vi "Check For License.vi"(8 "error in (no error)":errorcluster, 11 "VI Reference":refnum<vi>) -> (0 "Error Out":errorcluster, 2 "License Type":T1=enum."Professional", 3 "Valid License?":bool)   [LabVIEW 2022 SP3]
uses:
  <userlib>/_MGI/Error Reporter/MGI Error Reporter Base/MGI Error Reporter Base.lvclass
  Controls/License Types.ctl
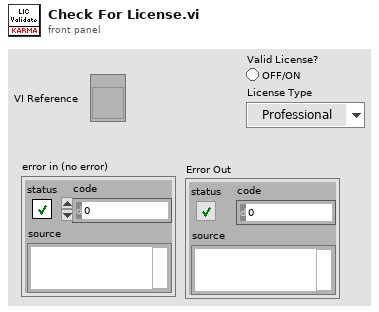
[diagram p1: front panel]
types:
  T1 = typedef "License Types.ctl" = enum16{"Evaluation", "Professional"}
  T2 = typedef "Paths.ctl" = cluster{"Configuration":path, "Event Logs":path, "Error Logs":path, "Configuration.ini":path}
  T3 = typedef "License File Data.ctl" = cluster{"Computer ID":string, "License Requested Date":string, "License Generated Date":string, "License Type":T1, "Evaluation Period":string, "License Generated Time":timestamp, "Sensor Serial Number":string}
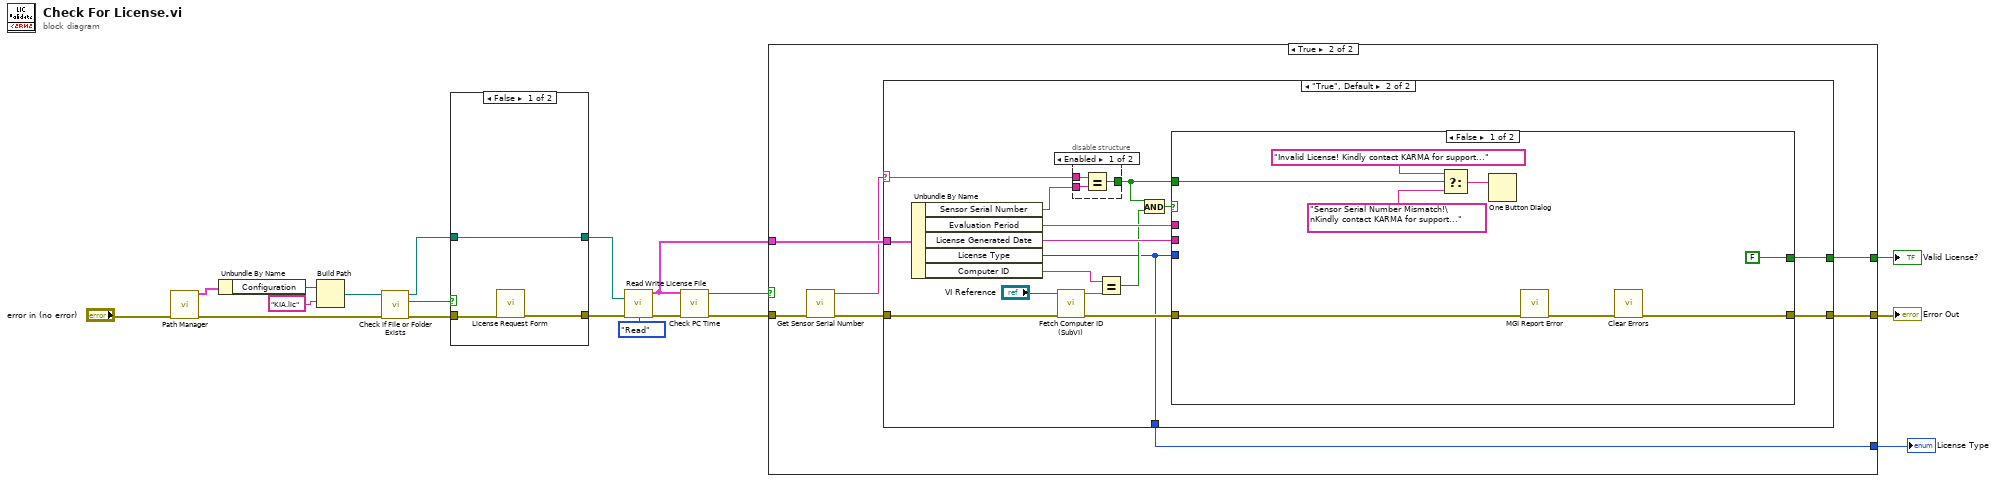
[diagram p0: block diagram]
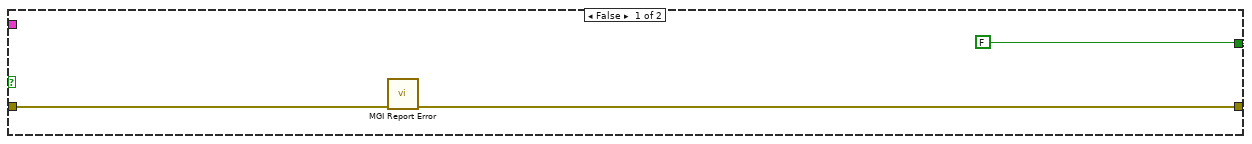
[diagram p2: hidden frame]
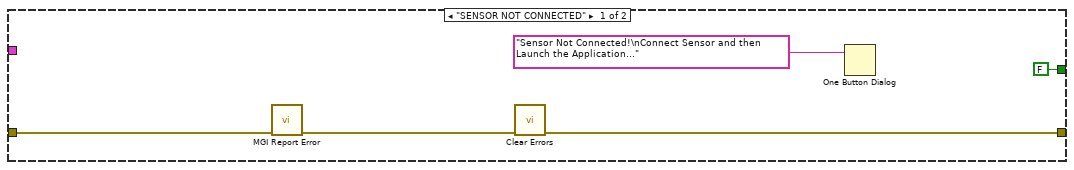
[diagram p3: hidden frame]
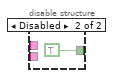
[diagram p4: hidden frame]
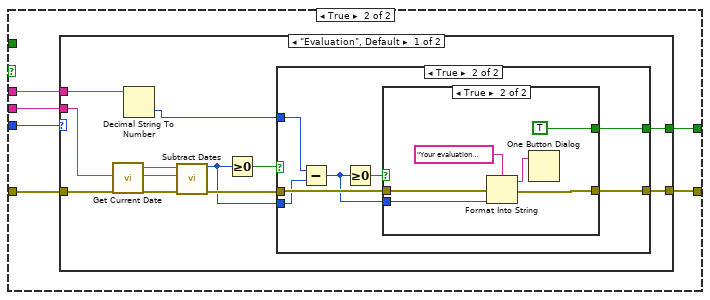
[diagram p5: hidden frame]
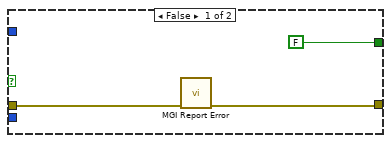
[diagram p6: hidden frame]
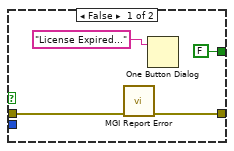
[diagram p7: hidden frame]
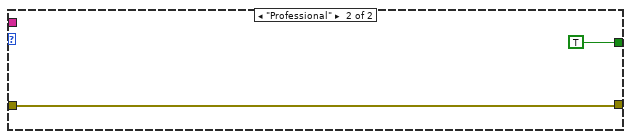
[diagram p8: hidden frame]
diagram:
  n1 = call "Path Manager.vi"("error in (no error)"="error in (no error)") -> ("Cluster"=w19:T2, "Error out"=w15:errorcluster)  [unwired: 13 in]
  n2 = Unbundle By Name(w19) -> ("Configuration"=w17:path)
  n3 = Build Path(base path=w17, name or relative path="KIA.lic") -> (appended path=w16:path)
  n4 = call <vilib>:"Check if File or Folder Exists.vi"("error in (no error)"=w15, "path"=w16) -> ("error out"=w13:errorcluster, "file or folder exists?"=w14:bool, "dup path"=w12:path)  [unwired: 7 in]
  n5 = case shown="False" w14 {
    tunnel: w13 -> [w22 w24]
    tunnel: w12 -> [w20 w23]
    tunnel: [w21 w24] -> w11
    tunnel: [w20 w23] -> w10
    frame False {
      n6 = call "License Request Form.vi"("Error in (no error)"=w22) -> ("Error out"=w21:errorcluster)  [unwired: 10 in]
    }
    frame True {
    }
  }
  n7 = call "Read Write License File.vi"("License File Path"=w10, "Error in (no error)"=w11, "Operation"=enum16{"Write", "Read"}."Read") -> ("License File Data Out"=w6:T3, "Error out"=w5:errorcluster)  [unwired: 10 in, 1 out]
  n8 = call "Check PC Time.vi"("Error in"=w5, "License File Data Out"=w6) -> ("Error out"=w4:errorcluster, "ValidTime?"=w2:bool)  [unwired: 8 in]
  n9 = case shown="True" w2 {
    tunnel: [_ w34] -> w8
    tunnel: w6 -> [_ w33]
    tunnel: w4 -> [w26 w30]
    tunnel: [w25 w32] -> w3
    tunnel: [FALSE w31] -> w1
    frame False {
      n10 = call <userlib>:"MGI Report Error.vi"("error in"=w26) -> ("no error"=w25:errorcluster)  [unwired: 10 in]
    }
    frame True {
      n11 = call "Get Sensor Serial Number.vi"("Error in (no error)"=w30) -> ("Error out"=w29:errorcluster, "Serial Number"=w28:string)  [unwired: 9 in]
      n12 = case shown="\"True\", Default" w28 {
        selector: w28 -> [_ w43]
        tunnel: [_ w40] -> w34
        tunnel: w33 -> [_ w49]
        tunnel: [w38 w48] -> w32
        tunnel: [FALSE w47] -> w31
        tunnel: w29 -> [w36 w44]
        frame "SENSOR NOT CONNECTED" {
          n13 = call <userlib>:"MGI Report Error.vi"("error in"=w36) -> ("no error"=w35:errorcluster)  [unwired: 10 in]
          n14 = call <vilib>:"Clear Errors.vi"("error in (no error)"=w35) -> ("error out"=w38:errorcluster)  [unwired: 5 in, 1 out]
          n15 = One Button Dialog(message="Sensor Not Connected!\nConnect Sensor and then Launch the Application...") -> ()  [unwired: 1 in, 1 out]
        }
        frame "True", Default {
          n16 = Unbundle By Name(w49) -> ("Sensor Serial Number"=w46:string, "Evaluation Period"=w51:string, "License Generated Date"=w52:string, "License Type"=w40:T1, "Computer ID"=w54:string)
          n17 = call "Fetch Computer ID (SubVI).vi"("Error in (no error)"=w44, "VI Reference"="VI Reference") -> ("Error out"=w53:errorcluster, "Computer ID"=w55:string)  [unwired: 8 in]
          n18 = disable-structure shown="Enabled" {
            disable-tunnel: w46 -> [w58 _]
            disable-tunnel: w43 -> [w57 _]
            disable-tunnel: [w56 TRUE] -> w41
            frame Enabled {
              n19 = Equal?(x=w57, y=w58) -> (x = y?=w56:bool)
            }
            frame Disabled {
            }
          }
          n20 = Equal?(x=w54, y=w55) -> (x = y?=w42:bool)
          n21 = And(x=w41, y=w42) -> (x .and. y?=w45:bool)
          n22 = case shown="False" w45 {
            tunnel: w53 -> [w61 w73]
            tunnel: w40 -> [_ w72]
            tunnel: w52 -> [_ w71]
            tunnel: [w62 w70] -> w48
            tunnel: w51 -> [_ w69]
            tunnel: [FALSE w68] -> w47
            tunnel: w41 -> [w66 _]
            frame False {
              n23 = Select(t="Invalid License! Kindly contact KARMA for support..." ("message"), s=w66, f="Sensor Serial Number Mismatch!\nKindly contact KARMA for support..." ("message")) -> (s? t:f=w64:string)
              n24 = One Button Dialog(message=w64) -> ()  [unwired: 1 in, 1 out]
              n25 = call <userlib>:"MGI Report Error.vi"("error in"=w61) -> ("no error"=w60:errorcluster)  [unwired: 10 in]
              n26 = call <vilib>:"Clear Errors.vi"("error in (no error)"=w60) -> ("error out"=w62:errorcluster)  [unwired: 5 in, 1 out]
            }
            frame True {
              n27 = case shown="\"Evaluation\", Default" w72 {
                tunnel: w73 -> [w83 w105]
                tunnel: w71 -> [w81 _]
                tunnel: [w77 w105] -> w70
                tunnel: w69 -> [w76 _]
                tunnel: [w74 TRUE] -> w68
                frame "Evaluation", Default {
                  n28 = call "Get Current Date.vi"() -> ("Date String"=w82:string)  [unwired: 8 in]
                  n29 = Decimal String To Number(string=w76) -> (number=w75:i32)  [unwired: 2 in, 1 out]
                  n30 = call "Subtract Dates.vi"("error in (no error)"=w83, "First date"=w81, "Second date"=w82) -> ("error out"=w79:errorcluster, "Elapsed days"=w78:i32)  [unwired: 7 in]
                  n31 = Greater Or Equal To 0?(x=w78) -> (x >= 0?=w80:bool)
                  n32 = case shown="True" w80 {
                    tunnel: w79 -> [w85 w93]
                    tunnel: w78 -> [_ w91]
                    tunnel: [w84 w92] -> w77
                    tunnel: w75 -> [_ w90]
                    tunnel: [FALSE w89] -> w74
                    frame False {
                      n33 = call <userlib>:"MGI Report Error.vi"("error in"=w85) -> ("no error"=w84:errorcluster)  [unwired: 10 in]
                    }
                    frame True {
                      n34 = Subtract(x=w90, y=w91) -> (x-y=w88:i32)
                      n35 = Greater Or Equal To 0?(x=w88) -> (x >= 0?=w87:bool)
                      n36 = case shown="True" w87 {
                        tunnel: w93 -> [w95 w103]
                        tunnel: [w94 w102] -> w92
                        tunnel: [FALSE TRUE] -> w89
                        tunnel: w88 -> [_ w100]
                        frame False {
                          n37 = call <userlib>:"MGI Report Error.vi"("error in"=w95) -> ("no error"=w94:errorcluster)  [unwired: 10 in]
                          n38 = One Button Dialog(message="License Expired...") -> ()  [unwired: 1 in, 1 out]
                        }
                        frame True {
                          n39 = Format Into String(format string="Your evaluation license will expire in %d days....", error in=w103, w100) -> (resulting string=w98:string, error out=w102:errorcluster)  [unwired: 1 in]
                          n40 = One Button Dialog(message=w98) -> ()  [unwired: 1 in, 1 out]
                        }
                      }
                    }
                  }
                }
                frame "Professional" {
                }
              }
            }
          }
        }
      }
    }
  }
  "Error Out" <- w3
  "Valid License?" <- w1
  "License Type" <- w8
